vi "Keithley 24XX Perform Limit Tests.vi"() -> ()   [LabVIEW 2018]
doc: "Performs limit tests on the device under test based on inputted settings."
uses:
  Keithley 24XX.lvlib
  Public/Data/Low Level/Fetch (Limit).vi
panel:
  in  "Source Mode  (0: Voltage)":u16(ring) items=["Voltage", "Current"]
  out "Limit Test Reading":dbl
  in  "Test 3 High Limit (1.5)":dbl=1.5
  in  "Test 3 Low Limit (0.5)":dbl=0.5
  in  "Test 2 High Limit (1)":dbl=2.0
  in  "Test 2 Low Limit (0)":dbl
  out "Test 3 Passed":bool
  out "Test 2 Passed":bool
  in  "Test Value Source  (0: Voltage)":u16(ring) items=["Voltage", "Current", "Resistance"]
  in  "VISA resource name":refnum<visa-resource-name>
  in  "Serial Configuration":T1={"Baud Rate"=9600, "Parity"=0, "Data Bits"=8, "Stop Bits"=10, "Flow Control"=0} {"Flow Control" items=["None", "XON/XOFF", "RTS/CTS", "XON/XOFF & RTS/CTS", "DTR/DSR", "XON/XOFF & DTR/DSR"]; "Stop Bits" items=["1.0"=10, "1.5"=15, "2.0"=20]; "Data Bits" items=["7"=7, "8"=8]; "Parity" items=["None", "Odd", "Even", "Mark", "Space"]; "Baud Rate" items=["300"=300, "600"=600, "1200"=1200, "2400"=2400, "4800"=4800, "9600"=9600, "19200"=19200]}
  in  "Output Level (.0001)":dbl=0.0001
  in  "Compliance  Level (10)":dbl=10.0
  # "(c) 2006 - 2015 National Instruments.  ALL RIGHTS RESERVED."
  # "Limit Test 2"
  # "Limit Test 3"
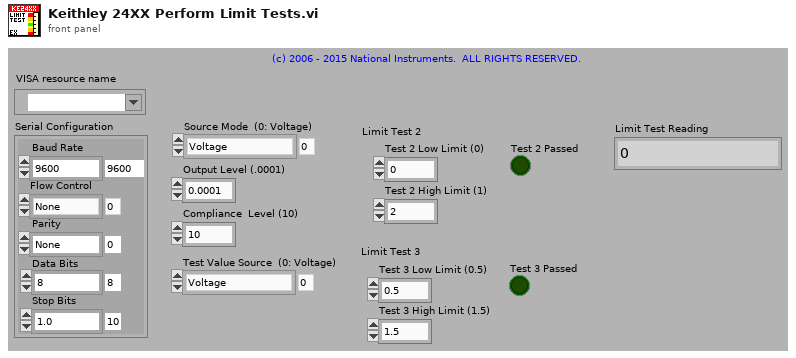
[diagram p1: front panel]
types:
  T1 = cluster{"Baud Rate":u32, "Parity":u16, "Data Bits":u16, "Stop Bits":u16, "Flow Control":u16}
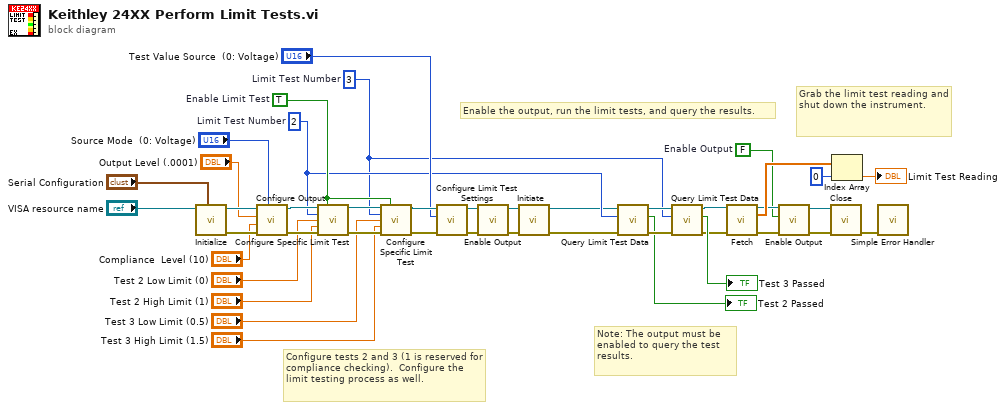
[diagram p0: block diagram]
diagram:
  w4 = FALSE  # Enable Output
  w34 = TRUE  # Enable Limit Test
  w23 = u16 3  # Limit Test Number
  w26 = u16 2  # Limit Test Number
  # "Grab the limit test reading and shut down the instrument."
  # "Note: The output must be enabled to query the test results."
  # "Enable the output, run the limit tests, and query the results."
  # "Configure tests 2 and 3 (1 is reserved for compliance checking).  Configure the limit testing process as well."
  n1 = call "Initialize.vi"("Serial Configuration"="Serial Configuration", "VISA resource name"="VISA resource name") -> ("error out"=w41:errorcluster, "VISA resource name out"=w42:refnum<visa-resource-name>)  [unwired: 8 in]
  n2 = call "Configure Output.vi"("Source Mode  (0: Voltage)"="Source Mode  (0: Voltage)", "error in (no error)"=w41, "Compliance  Level (0.1)"="Compliance  Level (10)", "Output Level (0)"="Output Level (.0001)", "VISA resource name"=w42) -> ("error out"=w35:errorcluster, "VISA resource name out"=w36:refnum<visa-resource-name>)  [unwired: 5 in]
  n3 = call "Configure Specific Limit Test.vi"("VISA resource name"=w36, "Enable Limit Test  (T:Enable)"=w34, "Limit Test Number (2)"=w26, "Low Limit (0)"="Test 2 Low Limit (0)", "High Limit (1)"="Test 2 High Limit (1)", "error in (no error)"=w35) -> ("VISA resource name out"=w38:refnum<visa-resource-name>, "error out"=w37:errorcluster)  [unwired: 8 in]
  n4 = call "Configure Specific Limit Test.vi"("VISA resource name"=w38, "Enable Limit Test  (T:Enable)"=w34, "Limit Test Number (2)"=w23, "Low Limit (0)"="Test 3 Low Limit (0.5)", "High Limit (1)"="Test 3 High Limit (1.5)", "error in (no error)"=w37) -> ("VISA resource name out"=w33:refnum<visa-resource-name>, "error out"=w32:errorcluster)  [unwired: 8 in]
  n5 = call "Configure Limit Test Settings.vi"("error in (no error)"=w32, "Test Value Source  (0: Voltage)"="Test Value Source  (0: Voltage)", "VISA resource name"=w33) -> ("error out"=w29:errorcluster, "VISA resource name out"=w30:refnum<visa-resource-name>)  [unwired: 7 in]
  n6 = call "Enable Output.vi"("error in (no error)"=w29, "VISA resource name"=w30) -> ("error out"=w28:errorcluster, "VISA resource name out"=w27:refnum<visa-resource-name>)  [unwired: 8 in]
  n7 = call "Initiate.vi"("error in (no error)"=w28, "VISA resource name"=w27) -> ("error out"=w10:errorcluster, "VISA resource name out"=w9:refnum<visa-resource-name>)  [unwired: 8 in]
  n8 = call "Query Limit Test Data.vi"("error in (no error)"=w10, "Test Number (2)"=w26, "VISA resource name"=w9) -> ("error out"=w25:errorcluster, "Test Passed"=→"Test 2 Passed":bool, "VISA resource name out"=w24:refnum<visa-resource-name>)  [unwired: 6 in]
  n9 = call "Query Limit Test Data.vi"("error in (no error)"=w25, "Test Number (2)"=w23, "VISA resource name"=w24) -> ("error out"=w14:errorcluster, "Test Passed"=→"Test 3 Passed":bool, "VISA resource name out"=w15:refnum<visa-resource-name>)  [unwired: 6 in]
  n10 = call-poly "Fetch.vi"("VISA resource name"=w15, "error in (no error)"=w14) -> ("VISA resource name out"=w6:refnum<visa-resource-name>, "Limit Test Readings"=w13:sgl[], "error out"=w5:errorcluster)  [unwired: 11 in]
  n11 = call "Enable Output.vi"("error in (no error)"=w5, "Enable Output (T: Enable)"=w4, "VISA resource name"=w6) -> ("error out"=w8:errorcluster, "VISA resource name out"=w7:refnum<visa-resource-name>)  [unwired: 7 in]
  n12 = call "Close.vi"("error in (no error)"=w8, "VISA resource name"=w7) -> ("error out"=w20:errorcluster)  [unwired: 9 in]
  n13 = Index Array(array=w13, index=0) -> (element=→"Limit Test Reading":sgl)
  n14 = call <vilib>:"Simple Error Handler.vi"("error in (no error)"=w20) -> ()  [unwired: 4 in, 5 out]
